vi "Var_GetReportingParameter.vi"(8 "error in":errorcluster, 10 "error code":i32, 11 "reporting params in":variant) -> (0 "error out":errorcluster, 1 "found?":bool, 2 "reporting parameter":T1, 3 "reporting params out":variant)   [LabVIEW 2013, in "CLM_ErrorHandler.lvlib" / "ErrorReporter.lvclass"]
uses:
  ErrorReporter.lvclass
  ReportingParameter.ctl
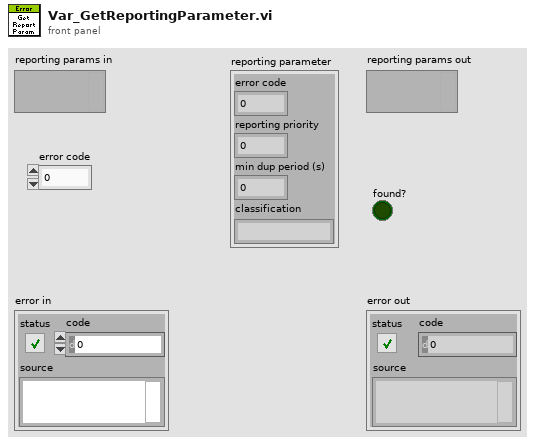
[diagram p1: front panel]
types:
  T1 = typedef "CLM_ErrorHandler.lvlib/ErrorReporter.lvclass/ReportingParameter.ctl" = cluster{"error code":i32, "reporting priority":i32, "min dup period (s)":dbl, "classification":string}
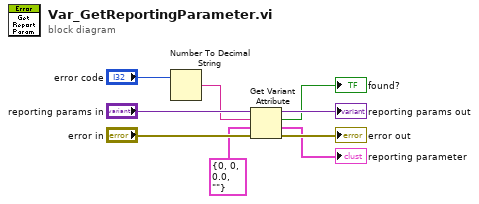
[diagram p0: block diagram]
diagram:
  n1 = Number To Decimal String(number="error code") -> (decimal integer string=w6:string)  [unwired: 1 in]
  n2 = Get Variant Attribute(Variant="reporting params in", name=w6, default value (empty Variant)=T1 {"error code"=0, "reporting priority"=0, "min dup period (s)"=0.0, "classification"=""} ("reporting parameter"), error in="error in") -> (duplicate Variant=→"reporting params out":variant, found=→"found?":bool, value=→"reporting parameter":T1, error out=→"error out":errorcluster)
